vi "Write(Command).vi"(6 "overwrite on timeout (T)":bool, 8 "error in (no error)":errorcluster, 9 "timeout in ms (0)":i32 format="%d ms", 10 "command":T1={"Command"=enum."Rx", "Command Parameters"={"arg1"=0, "arg2"=0}}, 11 "Transceiver Interface in":refnum<class "Transceiver Interface.lvclass">) -> (0 "error out":errorcluster, 1 "timed out?":bool, 3 "Transceiver Interface out":refnum<class "Transceiver Interface.lvclass">)   [LabVIEW 2017, in "DSF Core.lvlib" / "Transceiver Interface.lvclass"]
uses:
  Transceiver Interface.lvclass
  C:/github/data-sharing-framework/Data Sharing Framework/Source/Core/Engine/Classes/Interfaces/Interface/Interface.lvclass
  Command Data.ctl
  Command.ctl
  Command Parameters.ctl
  Interface/RT FIFO Data 16B.ctl
  Interface/RT FIFO Payload 16B.ctl
  Interface/Interface.lvclass/Interface.ctl
  Debug/FIFO Flags/FIFO Flags.lvclass/FIFO Flags.ctl
  Interface/Get Command FIFO.vi
  Interface/Write RT FIFO(16B).vi
  Interface/Get Debug Flags.vi
  Debug/FIFO Flags/Get Infinite Timeouts.vi
  Interface/Interface.lvclass
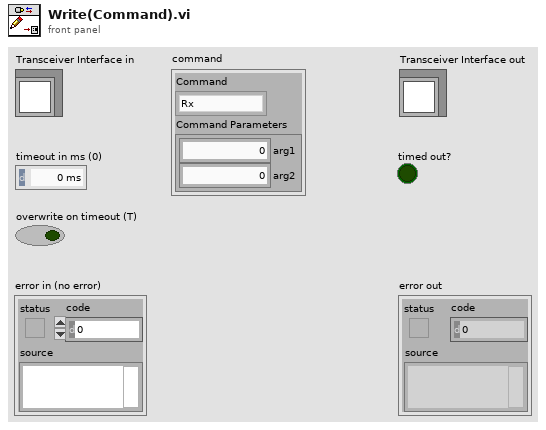
[diagram p1: front panel]
types:
  T1 = typedef "DSF Core.lvlib/Transceiver Interface.lvclass/Command Data.ctl" = cluster{"Command":T2, "Command Parameters":T3}
  T2 = typedef "DSF Core.lvlib/Transceiver Interface.lvclass/Command.ctl" = enum8{"Set Base Pointer", "Rx", "Tx", "Shutdown"}
  T3 = typedef "DSF Core.lvlib/Transceiver Interface.lvclass/Command Parameters.ctl" = cluster{"arg1":u64, "arg2":u64}
  T4 = typedef "DSF Core.lvlib/Interface.lvclass/RT FIFO Data 16B.ctl" = cluster{"Command":u8, "Payload":T5}
  T5 = typedef "DSF Core.lvlib/Interface.lvclass/RT FIFO Payload 16B.ctl" = cluster{"arg1":u64, "arg2":u64}
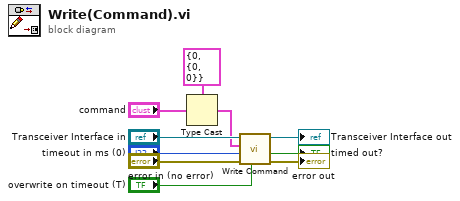
[diagram p0: block diagram]
diagram:
  n1 = Type Cast(type=T4 {"Command"=0, "Payload"={"arg1"=0, "arg2"=0}} ("element"), x="command") -> (*(type *) &x=w7:T4)
  n2 = call "Write Command.vi"("overwrite on timeout (T)"="overwrite on timeout (T)", "error in (no error)"="error in (no error)", "timeout in ms (0)"="timeout in ms (0)", "command"=w7, "Interface in"="Transceiver Interface in") -> ("error out"=→"error out":errorcluster, "timed out?"=→"timed out?":bool, "Interface out"=→"Transceiver Interface out":refnum<class "Transceiver Interface.lvclass">)  [unwired: 4 in]
